vi "Convert VCH to Card.vi"(11 "VCHList":T3) -> (3 "Card":T1={"Module Type"="", "Module Name"="", "ModuSN"="", "ModuIP"="", "Used?"=FALSE, "Connected"=FALSE, "Timing*"={"Sample Rate"=1000.0}, "Channels"=[]})   [LabVIEW 2016]
uses:
  Modules/DAQ-VirtualCH/SubVIs/VCH/Private/Ctrls/PSVCH_All Channels.ctl
  Modules/DAQ-Config/Controls/PSCHN_Card Para.ctl
  Modules/DAQ-Config/Controls/PSCHN_Channel Para.ctl
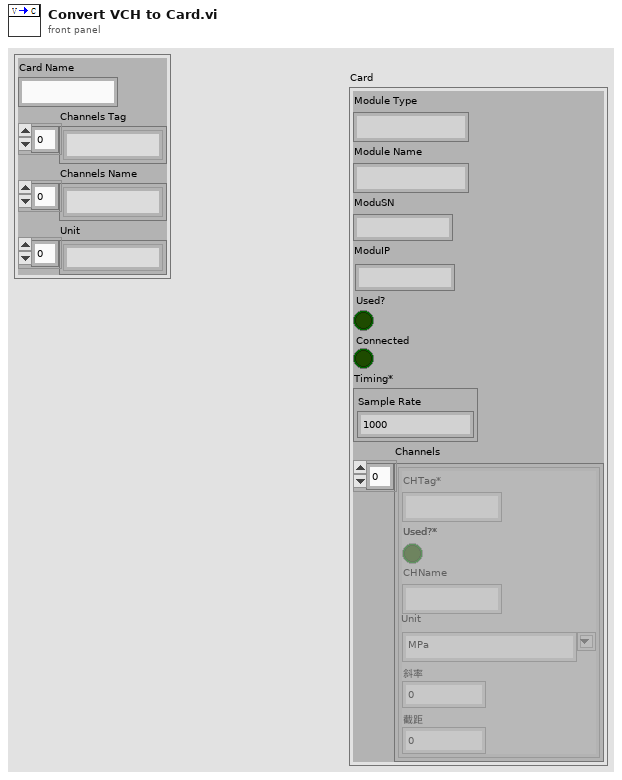
[diagram p1: front panel]
types:
  T1 = typedef "PSCHN_Card Para.ctl" = cluster{"Module Type":string, "Module Name":string, "ModuSN":string, "ModuIP":string, "Used?":bool, "Connected":bool, "Timing*":cluster{"Sample Rate":dbl}, "Channels":T2[]}
  T2 = typedef "PSCHN_Channel Para.ctl" = cluster{"CHTag*":string, "Used?*":bool, "CHName":string, "Unit":string, "斜率":dbl, "截距":dbl}
  T3 = typedef "PSVCH_All Channels.ctl" = cluster{"Card Name":string, "Channels Tag":string[], "Channels Name":string[], "Unit":string[]}
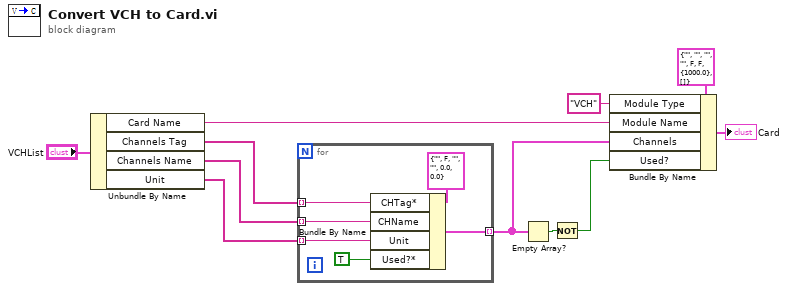
[diagram p0: block diagram]
diagram:
  n1 = Unbundle By Name("VCHList") -> ("Card Name"=w10:string, "Channels Tag"=w8:string[], "Channels Name"=w7:string[], "Unit"=w6:string[])
  n2 = for {
    tunnel: w8 -> [w16] mode=indexing
    tunnel: w7 -> [w15] mode=indexing
    tunnel: w6 -> [w13] mode=indexing
    tunnel: [w14] -> w3 mode=indexing
    n3 = Bundle By Name(cluster=T2 {"CHTag*"="", "Used?*"=FALSE, "CHName"="", "Unit"="", "斜率"=0.0, "截距"=0.0} ("Channel"), "CHTag*"=w16, "CHName"=w15, "Unit"=w13, "Used?*"=TRUE) -> (w14:T2)
  }
  n4 = Empty Array?(array=w3) -> (empty?=w2:bool)
  n5 = Not(x=w2) -> (.not. x?=w1:bool)
  n6 = Bundle By Name(cluster=T1 {"Module Type"="", "Module Name"="", "ModuSN"="", "ModuIP"="", "Used?"=FALSE, "Connected"=FALSE, "Timing*"={"Sample Rate"=1000.0}, "Channels"=[]} ("Card"), "Module Type"="VCH", "Module Name"=w10, "Channels"=w3, "Used?"=w1) -> (→"Card":T1)
